vi "absorptionImaging.vi"() -> ()   [LabVIEW 2009, in "run.lvlib"]
uses:
  testing/run.lvlib
  Tools/Filing/FileNeologist/FileNeologist.lvclass
panel:
  out "Images Taken":i32
  out "path":path
  in  "number of images":i32=3
  out "Image":T1(plugin-control)
  in  "Save":bool=TRUE
  out "Board Parameters":T2 {"Vertical bin" items=["1", "2"]; "Horizontal bin" items=["1", "2"]}
  in  "gain":i32(ring) items=["Low (X1)", "High (X2)"]
  in  "exp time":i32(slide)=300 min=1 max=10000 scale=0.0..300.0
  in  "V bin":i32(ring) items=["1", "2"]
  in  "H bin":i32(ring) items=["1", "2"]
  in  "trigger":bool=TRUE
  in  "Exposure mode":u16(ring) items=["Asynch shutter", "Double shot", "Video mode", "Auto exposure"]
  out "ccdtemp":i32(slide) scale=0.0..100.0
  in  "stop":bool
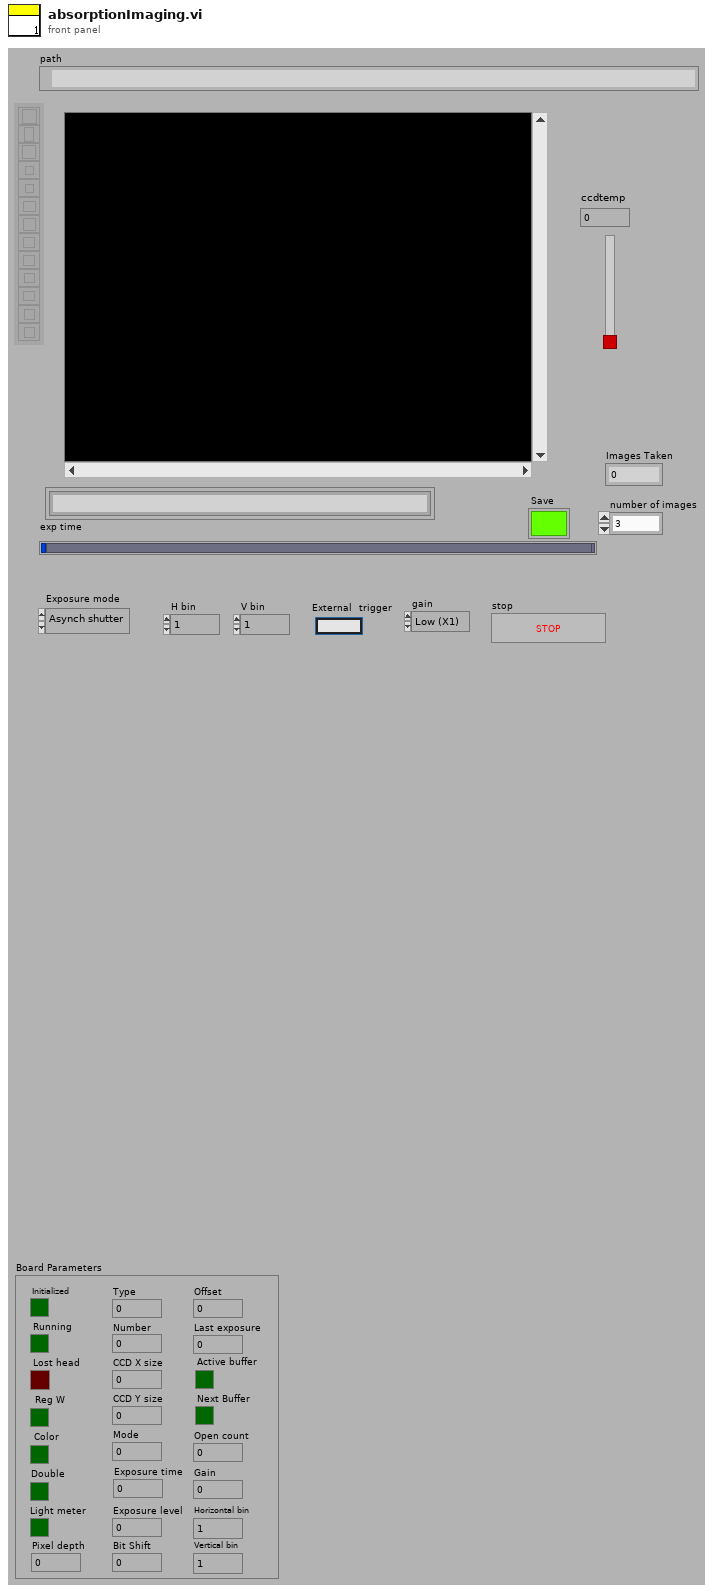
[diagram p1: front panel]
types:
  T1 = typedef "IMAQ Image.ctl" = refnum<image>
  T2 = cluster{"Type":u32, "Number":u32, "Initialized":bool, "Running":bool, "Lost head":bool, "CCD X size":u32, "CCD Y size":u32, "Mode":u32, "Exposure time":u32, "Exposure level":u32, "Horizontal bin":u32, "Vertical bin":u32, "Reg W":bool, "Gain":u32, "Pixel depth":i32, "Bit Shift":u32, "Offset":u32, "Last exposure":u32, "Double ":bool, "Light meter":bool, "Color":bool, "Open count":u32, "Active buffer":bool, "Next Buffer":bool}
  T3 = typedef "Image Type" = u32
  T4 = cluster{"ccdxsize":i32, "ccdy":i32, "pictx":i32, "picty":i32, "bitspixel":i32}
  T5 = cluster{"Write":bool, "Write done":bool, "Queued":bool, "Cancelled":bool, "Select":bool, "Select done":bool, "Burst":bool, "Size":bool, "Event":bool, "Timeout":bool, "Open":i32, "Map":i32, "Exposure":i32[], "Offset":i32[], "Size":i32[], "Transfer":i32[], "Total Size":i32}
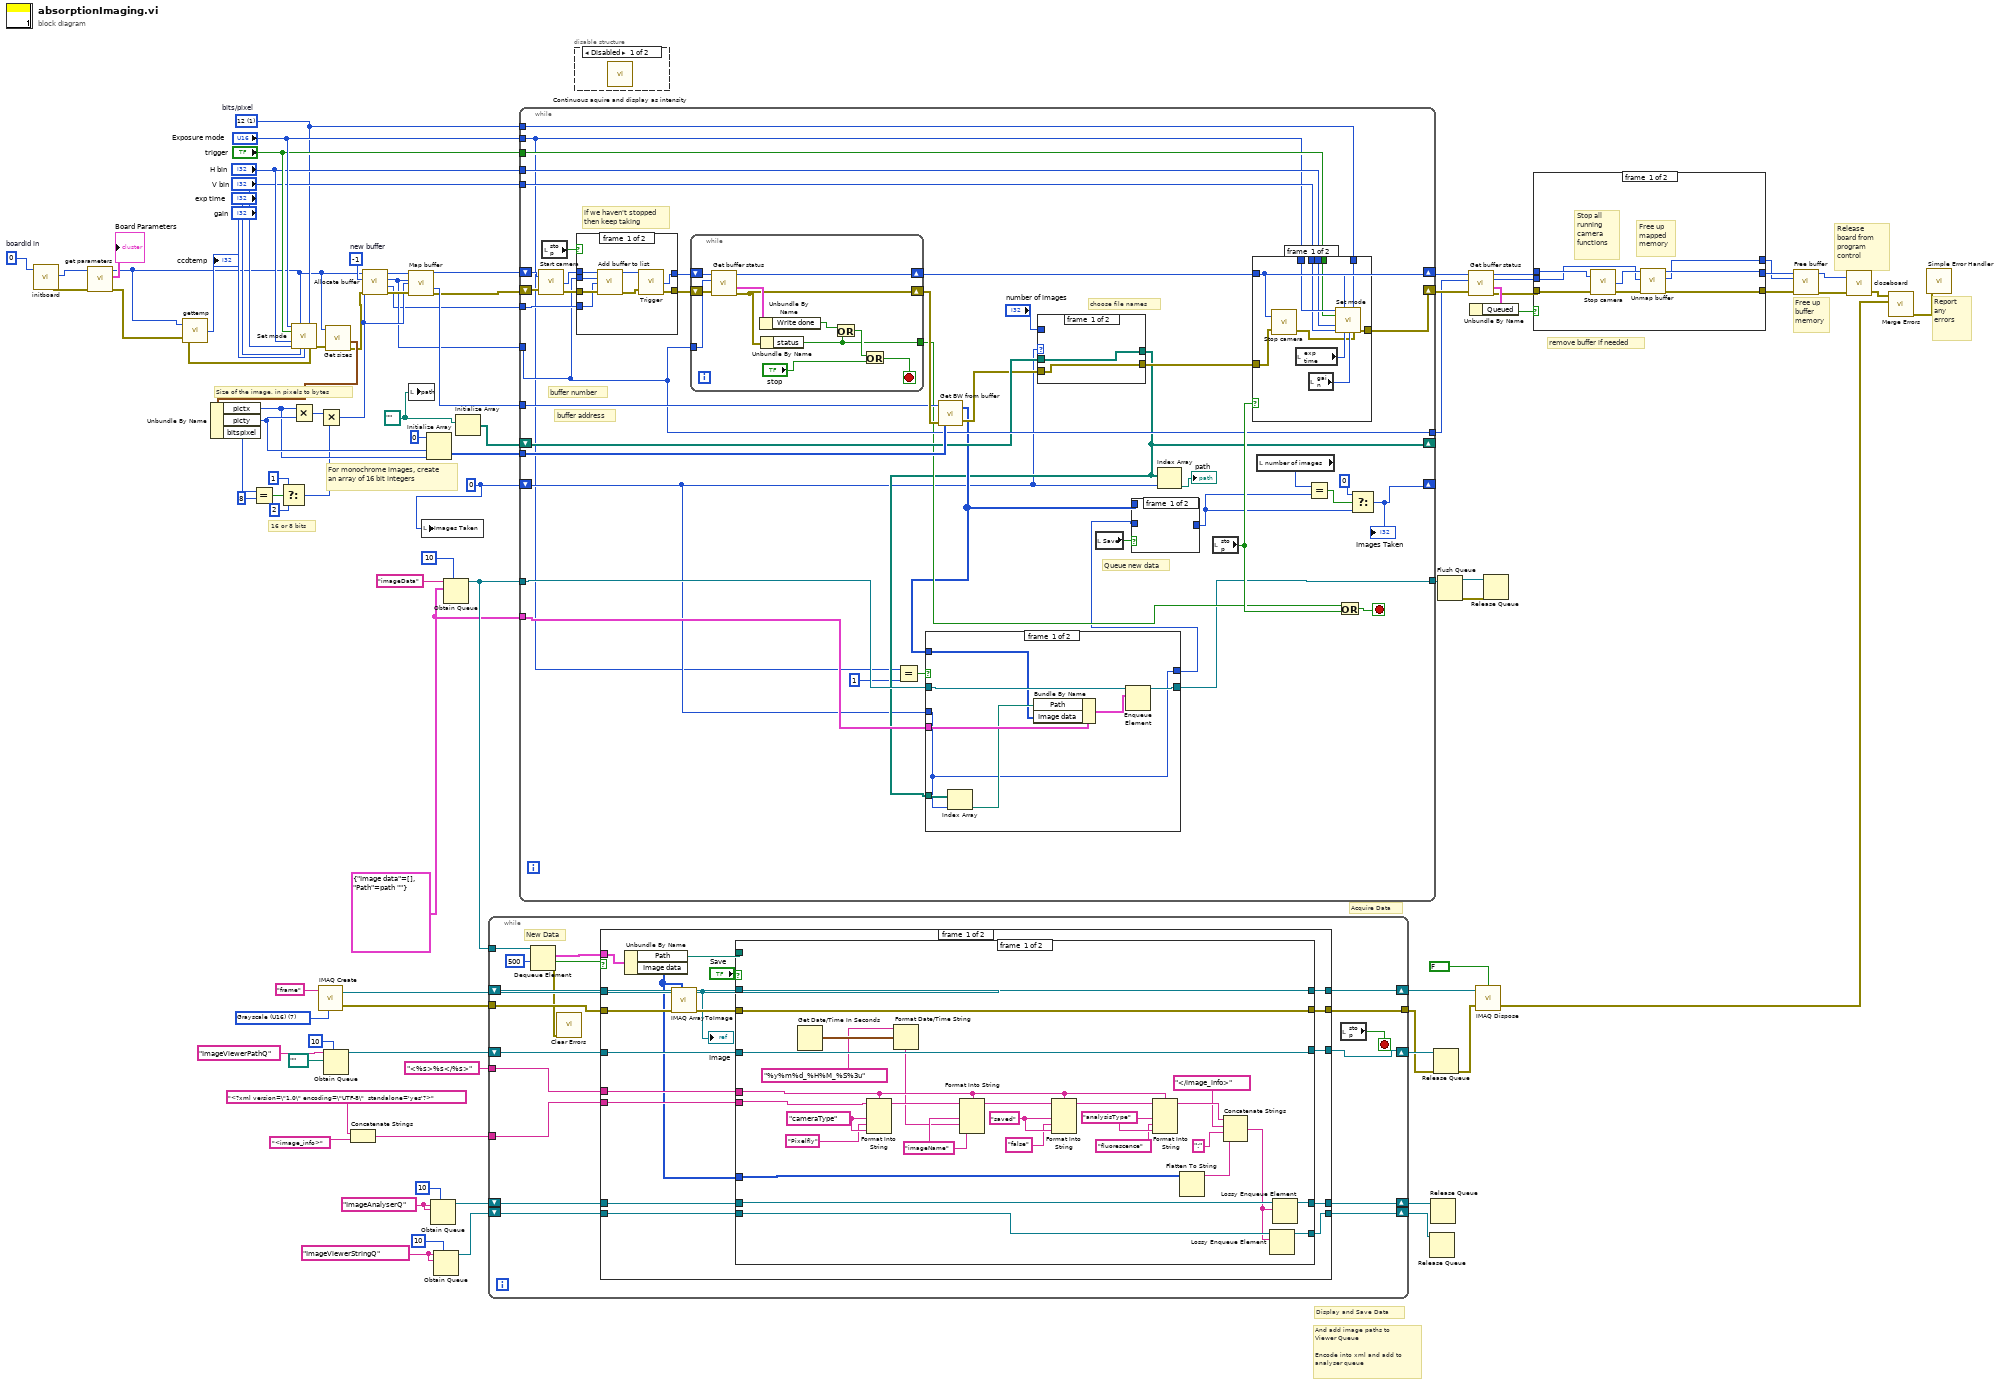
[diagram p0: block diagram]
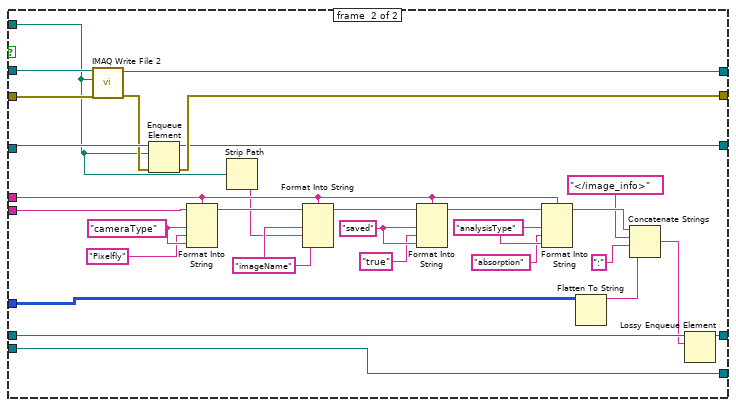
[diagram p2: hidden frame]
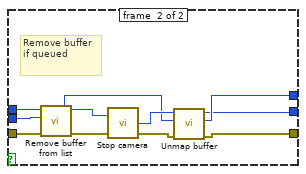
[diagram p5: hidden frame]
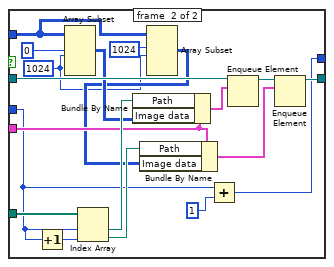
[diagram p6: hidden frame]
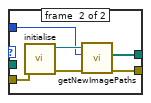
[diagram p7: hidden frame]
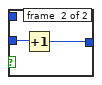
[diagram p8: hidden frame]
diagram:
  w11 = "ImageViewerStringQ"
  w15 = "ImageAnalyserQ"
  w27 = cluster{"Image data":u16[][], "Path":path} {"Image data"=[], "Path"=path ""}
  w36 = T3 7 items=["Grayscale (U8)", "Grayscale (I16)", "Grayscale (SGL)", "Complex (CSG)", "RGB (U32)", "HSL (U32)", "RGB (U64)", "Grayscale (U16)"] ("Image Type")
  w26 = path ""
  w25 = 0
  w55 = 1 items=["8", "12"]  # bits/pixel
  w71 = -1  # new buffer
  w75 = 0  # boardid in
  # "And add image paths to \nViewer Queue\n\nEncode into xml and add to\nanalyser queue"
  # "Acquire Data"
  # "Display and Save Data"
  # "remove buffer if needed"
  # "Report any errors"
  # "Release board from program control"
  # "Free up buffer memory"
  # "16 or 8 bits"
  # "For monochrome images, create an array of 16 bit integers"
  # "Size of the image, in pixels to bytes"
  n1 = call <instrlib>:"initboard.vi"("boardid in"=w75) -> ("boardid"=w87:i32, "error out"=w45:errorcluster)  [unwired: 3 in, 1 out]
  n2 = call <instrlib>:"get parameters.vi"("error in (no error)"=w45, "Handle in"=w87) -> ("error out"=w4:errorcluster, "Board Parameters"=→"Board Parameters":T2, "Error out"=w1:i32)  [unwired: 2 in, 1 out]
  n3 = call <instrlib>:"gettemp.vi"("Handle in"=w1, "error in (no error)"=w4) -> ("ccdtemp"=→"ccdtemp":i32, "error out"=w88:errorcluster)  [unwired: 1 out]
  n4 = call <instrlib>:"Set mode.vi"("Exposure mode"="Exposure mode", "Handle in"=w1, "bits/pixel"=w55, "trigger"="trigger", "H bin"="H bin", "V bin"="V bin", "exp time"="exp time", "gain"="gain", "error in (no error)"=w88) -> ("error out"=w3:errorcluster)  [unwired: 6 in]
  n5 = call "IMAQ Create"("Image Name"="frame", "Image Type"=w36) -> ("New Image"=w35:T1, "error out"=w34:errorcluster)  [unwired: 3 in]
  n6 = Obtain Queue(max queue size (-1, unlimited)=10, name (unnamed)="ImageViewerPathQ", element data type=path "") -> (queue out=w23:refnum<queue>)  [unwired: 2 in, 2 out]
  n7 = call <instrlib>:"Get sizes.vi"("Handle in"=w1, "error in (no error)"=w3) -> ("Picture parameters"=w83:T4, "error out"=w2:errorcluster)  [unwired: 1 in, 2 out]
  n8 = Unbundle By Name(w83) -> ("pictx"=w80:i32, "picty"=w81:i32, "bitspixel"=w82:i32)
  n9 = Equal?(x=w82, y=8) -> (x = y?=w79:bool)
  n10 = Select(t=1, s=w79, f=2) -> (s? t:f=w76:i32)
  n11 = Multiply(x=w80, y=w81) -> (x*y=w39:i32)
  n12 = Multiply(x=w39, y=w76) -> (x*y=w73:i32)
  n13 = Concatenate Strings("<?xml version=\"1.0\" encoding=\"UTF-8\"  standalone='yes'?>", "<image_info>") -> (w17:string)
  n14 = call <instrlib>:"Allocate buffer.vi"("error in (no error)"=w2, "Size request"=w73, "Buffer request"=w71, "Handle in"=w1) -> ("error out"=w86:errorcluster, "Size"=w53:i32, "Buffer number"=w54:i32, "Handle out"=w89:i32)
  n15 = call <instrlib>:"Map buffer.vi"("Handle in"=w89, "Buffer in"=w54, "size"=w73, "error in (no error)"=w86) -> ("Handle out"=w52:i32, "Buffer address"=w74:i32, "error out"=w51:errorcluster)  [unwired: 8 in, 1 out]
  n16 = local write "path"(w26) -> ()
  n17 = local write "Images Taken"(w25) -> ()
  n18 = Initialize Array(u16 0 ("16 bit integers"), w81, w80) -> (w72:u16[][])
  n19 = Obtain Queue(max queue size (-1, unlimited)=10, name (unnamed)=w15, element data type=w15) -> (queue out=w14:refnum<queue>)  [unwired: 2 in, 2 out]
  n20 = Obtain Queue(max queue size (-1, unlimited)=10, name (unnamed)=w11, element data type=w11) -> (queue out=w12:refnum<queue>)  [unwired: 2 in, 2 out]
  n21 = Obtain Queue(max queue size (-1, unlimited)=10, name (unnamed)="imageData", element data type=w27) -> (queue out=w32:refnum<queue>)  [unwired: 2 in, 2 out]
  n22 = Initialize Array(w26) -> (w38:path[])  [unwired: 1 in]
  n23 = while {
    tunnel: w34 -> [w106]
    tunnel: [w104] -> w21
    tunnel: w32 -> [w102]
    shift-right: [w96] -> w22
    shift-left: w23 -> [w97]
    shift-right: [w105] -> w33
    shift-left: w35 -> [w107]
    tunnel: w17 -> [w95]
    tunnel: "<%s>%s</%s>" -> [w94]
    shift-right: [w92] -> w13
    shift-left: w14 -> [w93]
    shift-right: [w90] -> w10
    shift-left: w12 -> [w91]
    stop <- w103 stop-if-true
    # "New Data"
    n24 = Dequeue Element(queue=w102, timeout in ms (-1)=500) -> (element=w101:cluster{"Image data":u16[][], "Path":path}, timed out?=w100:bool, error out=w98:errorcluster)  [unwired: 1 in, 1 out]
    n25 = call <vilib>:"Clear Errors.vi"("error in (no error)"=w98) -> ()  [unwired: 6 in, 1 out]
    n26 = case shown="False" w100 {
      tunnel: w107 -> [w124 w188]
      tunnel: w106 -> [w123 w187]
      tunnel: [w120 w188] -> w105
      tunnel: [w119 w187] -> w104
      tunnel: w101 -> [w118 _]
      tunnel: w97 -> [w116 w186]
      tunnel: [w115 w186] -> w96
      tunnel: w95 -> [w113 _]
      tunnel: w94 -> [w114 _]
      tunnel: w93 -> [w112 w185]
      tunnel: [w111 w185] -> w92
      tunnel: w91 -> [w110 w184]
      tunnel: [w109 w184] -> w90
      frame #0 {
        n27 = Unbundle By Name(w118) -> ("Path"=w117:path, "Image data"=w108:u16[][])
        n28 = call "IMAQ ArrayToImage"("Image Pixels (U16)"=w108, "error in (no error)"=w123, "Image"=w124) -> ("error out"=w125:errorcluster, "Image Out"=w122:T1)  [unwired: 7 in]
        "Image" <- w122
        n29 = case shown="True" "Save" {
          tunnel: [w153 w183] -> w120
          tunnel: [w152 w178] -> w119
          tunnel: w125 -> [w152 w182]
          tunnel: w122 -> [w153 w181]
          tunnel: w117 -> [_ w164]
          tunnel: w116 -> [w151 w180]
          tunnel: [w151 w177] -> w115
          tunnel: w114 -> [w135 w166]
          tunnel: w113 -> [w134 w165]
          tunnel: w108 -> [w133 w159]
          tunnel: w112 -> [w150 w157]
          tunnel: [w127 w155] -> w111
          tunnel: w110 -> [w129 w154]
          tunnel: [w128 w154] -> w109
          frame #0 {
            w147 = "analysisType"
            w145 = "saved"
            w141 = "imageName" ("Key")
            w140 = "cameraType"
            n30 = Get Date/Time In Seconds() -> (seconds since 1Jan1904=w132:timestamp)
            n31 = Format Into String(format string=w135, initial string=w134, w140, "Pixelfly", w140) -> (resulting string=w143:string)  [unwired: 1 in, 1 out]
            n32 = Format Date/Time String(time format string (%c)="%y%m%d_%H%M_%S%3u", seconds (now)=w132) -> (date/time string=w130:string)  [unwired: 1 in]
            n33 = Format Into String(format string=w135, initial string=w143, w141, w130, w141) -> (resulting string=w144:string)  [unwired: 1 in, 1 out]
            n34 = Format Into String(format string=w135, initial string=w144, w145, "false", w145) -> (resulting string=w148:string)  [unwired: 1 in, 1 out]
            n35 = Format Into String(format string=w135, initial string=w148, w147, "fluorescence", w147) -> (resulting string=w149:string)  [unwired: 1 in, 1 out]
            n36 = Flatten To String(anything=w133) -> (data string=w136:string)  [unwired: 3 in, 2 out]
            n37 = Concatenate Strings(w149, "</image_info>", ":", w136) -> (w126:string)
            n38 = Lossy Enqueue Element(queue=w129, element=w126) -> (queue out=w128:refnum<queue>)  [unwired: 1 in, 3 out]
            n39 = Lossy Enqueue Element(queue=w150, element=w126) -> (queue out=w127:refnum<queue>)  [unwired: 1 in, 3 out]
          }
          frame #1 {
            w174 = "analysisType"
            w172 = "saved"
            w168 = "imageName" ("Key")
            w167 = "cameraType"
            n40 = call-poly "IMAQ Write File 2"("error in (no error)"=w182, "File Path"=w164, "Image"=w181) -> ("error out"=w179:errorcluster, "Image Out (duplicate)"=w183:T1)  [unwired: 7 in]
            n41 = Enqueue Element(queue=w180, element=w164, error in (no error)=w179) -> (queue out=w177:refnum<queue>, error out=w178:errorcluster)  [unwired: 1 in, 1 out]
            n42 = Format Into String(format string=w166, initial string=w165, w167, "Pixelfly", w167) -> (resulting string=w170:string)  [unwired: 1 in, 1 out]
            n43 = Strip Path(path=w164) -> (name=w163:string)  [unwired: 1 out]
            n44 = Format Into String(format string=w166, initial string=w170, w168, w163, w168) -> (resulting string=w171:string)  [unwired: 1 in, 1 out]
            n45 = Format Into String(format string=w166, initial string=w171, w172, "true", w172) -> (resulting string=w175:string)  [unwired: 1 in, 1 out]
            n46 = Format Into String(format string=w166, initial string=w175, w174, "absorption", w174) -> (resulting string=w176:string)  [unwired: 1 in, 1 out]
            n47 = Flatten To String(anything=w159) -> (data string=w158:string)  [unwired: 3 in, 2 out]
            n48 = Concatenate Strings(w176, "</image_info>", ":", w158) -> (w156:string)
            n49 = Lossy Enqueue Element(queue=w157, element=w156) -> (queue out=w155:refnum<queue>)  [unwired: 1 in, 3 out]
          }
        }
      }
      frame #1 {
      }
    }
    n50 = local read "stop"() -> (w103:bool)
  }
  n51 = while {
    tunnel: w54 -> [w212]
    shift-right: [w217] -> w66
    shift-left: w52 -> [w216]
    shift-right: [w218] -> w65
    shift-left: w51 -> [w211]
    tunnel: w74 -> [w226]
    tunnel: w72 -> [w225]
    tunnel: "Exposure mode" -> [w189]
    tunnel: "trigger" -> [w221]
    tunnel: "H bin" -> [w220]
    tunnel: "V bin" -> [w219]
    tunnel: w55 -> [w222]
    tunnel: w53 -> [w224]
    tunnel: [w212] -> w49
    shift-right: [w210] -> _
    shift-left: w25 -> [w190]
    shift-right: [w194] -> _
    shift-left: w38 -> [w206]
    tunnel: w32 -> [w199]
    tunnel: [w196] -> w28
    tunnel: w27 -> [w195]
    stop <- w223 stop-if-true
    # "Queue new data"
    # "choose file names"
    # "buffer address"
    # "buffer number"
    # "if we haven't stopped\nthen keep taking"
    n52 = call <instrlib>:"Start camera.vi"("Handle in"=w216, "error in (no error)"=w211) -> ("Handle out"=w215:i32, "error out"=w214:errorcluster)  [unwired: 1 out]
    n53 = local read "stop"() -> (w230:bool)
    n54 = case shown="False" w230 {
      tunnel: w214 -> [w287 w288]
      tunnel: [w285 w288] -> w229
      tunnel: w215 -> [w284 w289]
      tunnel: [w282 w289] -> w228
      tunnel: w212 -> [w281 _]
      tunnel: w224 -> [w280 _]
      frame #0 {
        n55 = call <instrlib>:"Add buffer to list.vi"("Handle in"=w284, "Buffer in"=w281, "size"=w280, "error in (no error)"=w287) -> ("Handle out"=w283:i32, "error out"=w286:errorcluster)  [unwired: 9 in, 1 out]
        n56 = call <instrlib>:"Trigger.vi"("Handle in"=w283, "error in (no error)"=w286) -> ("Handle out"=w282:i32, "error out"=w285:errorcluster)  [unwired: 1 out]
      }
      frame #1 {
      }
    }
    n57 = while {
      tunnel: w212 -> [w293]
      shift-right: [w291] -> w217
      shift-left: w228 -> [w294]
      shift-right: [w292] -> w227
      shift-left: w229 -> [w295]
      tunnel: [w290] -> w200
      stop <- w296 stop-if-true
      n58 = call <instrlib>:"Get buffer status.vi"("error in (no error)"=w295, "Buffer request"=w293, "Handle in"=w294) -> ("error out"=w292:errorcluster, "Buffer status"=w300:T5, "Handle out"=w291:i32)  [unwired: 1 in, 1 out]
      n59 = Unbundle By Name(w300) -> ("Write done"=w299:bool)
      n60 = Unbundle By Name(w292) -> ("status"=w290:bool)
      n61 = Or(x=w299, y=w290) -> (x .or. y?=w298:bool)
      n62 = Or(x=w298, y="stop") -> (x .or. y?=w296:bool)
    }
    n63 = Equal?(x=w189, y=1) -> (x = y?=w193:bool)
    n64 = call <instrlib>:"Get BW from buffer.vi"("error in (no error)"=w227, "Array input"=w225, "Buffer address"=w226) -> ("error out"=w205:errorcluster, "Image data"=w198:u16[][])
    n65 = case shown="0" w190 {
      tunnel: [w259 w263] -> w194
      tunnel: w206 -> [w259 _]
      tunnel: w205 -> [w258 w262]
      tunnel: [w258 w261] -> w201
      tunnel: "number of images" -> [_ w260]
      frame #0 {
      }
      frame #1 {
        n66 = call "initialise.vi"("error in (no error)"=w262) -> ("error out"=w264:errorcluster, "FileNeologist out"=w265:refnum<class "FileNeologist.lvclass">)  [unwired: 9 in]
        n67 = call "getNewImagePaths.vi"("error in (no error)"=w264, "numberOfImages"=w260, "FileNeologist in"=w265) -> ("error out"=w261:errorcluster, "Paths"=w263:path[])  [unwired: 6 in, 1 out]
      }
    }
    n68 = case shown="True" w193 {
      tunnel: w199 -> [w237 w257]
      tunnel: [w238 w244] -> w196
      tunnel: w195 -> [w236 w248]
      tunnel: w198 -> [w233 w254]
      tunnel: w194 -> [w235 w252]
      tunnel: w190 -> [w231 w242]
      tunnel: [w231 w240] -> w191
      frame #0 {
        n69 = Index Array(array=w235, index=w231) -> (element=w234:path)
        n70 = Bundle By Name(cluster=w236, "Path"=w234, "Image data"=w233) -> (w232:cluster{"Image data":u16[][], "Path":path})
        n71 = Enqueue Element(queue=w237, element=w232) -> (queue out=w238:refnum<queue>)  [unwired: 2 in, 2 out]
      }
      frame #1 {
        w239 = 1024
        n72 = Increment(x=w242) -> (x+1=w251:i32)
        n73 = Array Subset(array=w254, index (row)=0, length (row)=w239) -> (w249:u16[][])  [unwired: 2 in]
        n74 = Index Array(array=w252, index #1=w242, index #2=w251) -> (element #1=w250:path, element #2=w247:path)
        n75 = Bundle By Name(cluster=w248, "Path"=w250, "Image data"=w249) -> (w256:cluster{"Image data":u16[][], "Path":path})
        n76 = Array Subset(array=w254, index (row)=1024, length (row)=w239) -> (w246:u16[][])  [unwired: 2 in]
        n77 = Bundle By Name(cluster=w248, "Path"=w247, "Image data"=w246) -> (w243:cluster{"Image data":u16[][], "Path":path})
        n78 = Add(x=w242, y=1) -> (x+y=w240:i32)
        n79 = Enqueue Element(queue=w257, element=w256) -> (queue out=w245:refnum<queue>)  [unwired: 2 in, 2 out]
        n80 = Enqueue Element(queue=w245, element=w243) -> (queue out=w244:refnum<queue>)  [unwired: 2 in, 2 out]
      }
    }
    n81 = local read "Save"() -> (w202:bool)
    n82 = case shown="True" w202 {
      tunnel: w191 -> [_ w267]
      tunnel: [_ w266] -> w208
      tunnel: w198 -> [_ _]
      frame #0 {
      }
      frame #1 {
        n83 = Increment(x=w267) -> (x+1=w266:i32)
      }
    }
    n84 = Index Array(array=w194, index=w190) -> (element=→"path":path)
    n85 = local read "stop"() -> (w213:bool)
    n86 = case shown="False" w213 {
      tunnel: w222 -> [w278 _]
      tunnel: w189 -> [w277 _]
      tunnel: w221 -> [w276 _]
      tunnel: w220 -> [w275 _]
      tunnel: w219 -> [w274 _]
      tunnel: [w271 w279] -> w218
      tunnel: w217 -> [w269 _]
      tunnel: w201 -> [w268 w279]
      frame #0 {
        n87 = call <instrlib>:"Stop camera.vi"("Handle in"=w269, "error in (no error)"=w268) -> ("error out"=w270:errorcluster)  [unwired: 2 out]
        n88 = local read "exp time"() -> (w273:i32)
        n89 = local read "gain"() -> (w272:i32)
        n90 = call <instrlib>:"Set mode.vi"("Exposure mode"=w277, "Handle in"=w269, "bits/pixel"=w278, "trigger"=w276, "H bin"=w275, "V bin"=w274, "exp time"=w273, "gain"=w272, "error in (no error)"=w270) -> ("error out"=w271:errorcluster)  [unwired: 6 in]
      }
      frame #1 {
      }
    }
    n91 = local read "number of images"() -> (w203:i32)
    n92 = Equal?(x=w203, y=w208) -> (x = y?=w209:bool)
    n93 = Or(x=w200, y=w213) -> (x .or. y?=w223:bool)
    n94 = Select(t=0, s=w209, f=w208) -> (s? t:f=w210:i32)
    "Images Taken" <- w210
  }
  n95 = disable-structure shown="Disabled" {
    frame #0 {
      n96 = call <instrlib>:"Continuous aquire and display as intensity.vi"() -> ()  [unwired: 1 in]
    }
    frame #1 {
    }
  }
  n97 = Release Queue(queue=w10) -> ()  [unwired: 2 in, 3 out]
  n98 = Release Queue(queue=w13) -> ()  [unwired: 2 in, 3 out]
  n99 = Release Queue(queue=w22, error in (no error)=w21) -> (error out=w20:errorcluster)  [unwired: 1 in, 2 out]
  n100 = Flush Queue(queue=w28) -> (queue out=w30:refnum<queue>, error out=w29:errorcluster)  [unwired: 1 in, 1 out]
  n101 = call <instrlib>:"Get buffer status.vi"("error in (no error)"=w65, "Buffer request"=w49, "Handle in"=w66) -> ("error out"=w67:errorcluster, "Buffer status"=w68:T5, "Buffer number"=w64:i32, "Handle out"=w63:i32)  [unwired: 1 in]
  n102 = Unbundle By Name(w68) -> ("Queued"=w50:bool)
  n103 = call "IMAQ Dispose"("All Images? (No)"=FALSE, "Image"=w33, "error in (no error)"=w20) -> ("error out"=w41:errorcluster)  [unwired: 3 in]
  n104 = Release Queue(queue=w30, error in (no error)=w29) -> ()  [unwired: 1 in, 3 out]
  n105 = case shown="True" w50 {
    tunnel: w67 -> [w305 w319]
    tunnel: [w303 w309] -> w46
    tunnel: w64 -> [w304 w318]
    tunnel: w63 -> [w306 w317]
    tunnel: [w302 w310] -> w48
    tunnel: [w301 w311] -> w47
    frame #0 {
      # "Free up mapped memory"
      # "Stop all running camera functions"
      n106 = call <instrlib>:"Stop camera.vi"("Handle in"=w306, "error in (no error)"=w305) -> ("Handle out"=w308:i32, "error out"=w307:errorcluster)  [unwired: 1 out]
      n107 = call <instrlib>:"Unmap buffer.vi"("error in (no error)"=w307, "Buffer in"=w304, "Handle in"=w308) -> ("error out"=w303:errorcluster, "Buffer number"=w301:i32, "Handle out"=w302:i32)  [unwired: 2 in]
    }
    frame #1 {
      # "Remove buffer if queued"
      n108 = call <instrlib>:"Remove buffer from list.vi"("error in (no error)"=w319, "Buffer in"=w318, "Handle in"=w317) -> ("error out"=w316:errorcluster, "Buffer number"=w312:i32, "Handle out"=w315:i32)  [unwired: 2 in]
      n109 = call <instrlib>:"Stop camera.vi"("Handle in"=w315, "error in (no error)"=w316) -> ("Handle out"=w313:i32, "error out"=w314:errorcluster)  [unwired: 1 out]
      n110 = call <instrlib>:"Unmap buffer.vi"("error in (no error)"=w314, "Buffer in"=w312, "Handle in"=w313) -> ("error out"=w309:errorcluster, "Buffer number"=w311:i32, "Handle out"=w310:i32)  [unwired: 2 in]
    }
  }
  n111 = call <instrlib>:"Free buffer.vi"("error in (no error)"=w46, "Buffer in"=w47, "Handle in"=w48) -> ("error out"=w69:errorcluster, "Handle out"=w62:i32)  [unwired: 2 in, 1 out]
  n112 = call <instrlib>:"closeboard.vi"("Handle in"=w62, "error in (no error)"=w69) -> ("error out"=w43:errorcluster)  [unwired: 2 out]
  n113 = call <vilib>:"Merge Errors.vi"("error in 2 (no error)"=w41, "error in 1 (no error)"=w43) -> ("error out"=w42:errorcluster)  [unwired: 5 in]
  n114 = call <vilib>:"Simple Error Handler.vi"("error in (no error)"=w42) -> ()  [unwired: 4 in, 5 out]
